vi "RIMAS Detector Send Command.vi"(8 "Error In":errorcluster, 10 "Command":string, 11 "Detector Ref":refnum<k5>) -> (0 "Error Out":errorcluster, 2 "Sent String":string, 3 "Detector Ref dup":refnum<k5>)   [LabVIEW 2021]
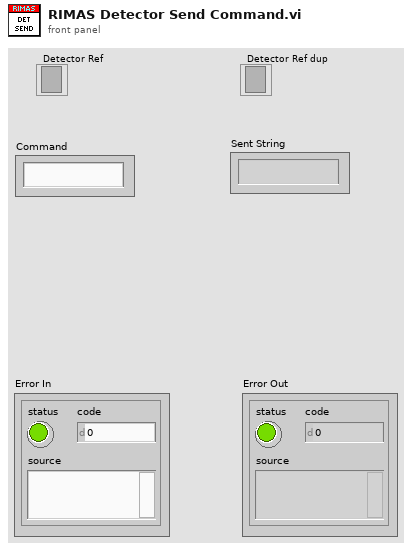
[diagram p1: front panel]
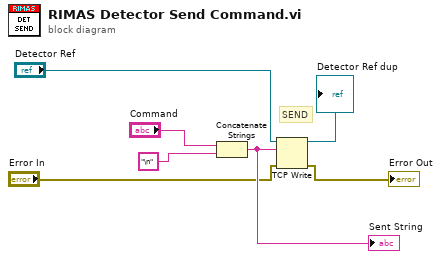
[diagram p0: block diagram]
diagram:
  # "SEND"
  n1 = Concatenate Strings("Command", "\n") -> (w7:string)
  "Sent String" <- w7
  n2 = TCP Write(connection ID="Detector Ref", data in=w7, error in (no error)="Error In") -> (connection ID out=→"Detector Ref dup":refnum<k5>, error out=→"Error Out":errorcluster)  [unwired: 1 in, 1 out]
